vi "Subvi MultiMode Image.vi"(2 "ImageRepeatNum":u32, 3 "InFileName":string) -> (0 "ImgAbort":bool, 1 "ImgTaken":bool)   [LabVIEW 2012]
uses:
  ProSCI Global.vi
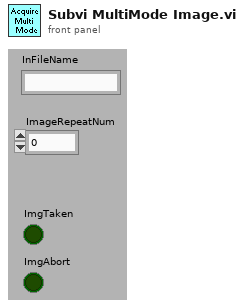
[diagram p1: front panel]
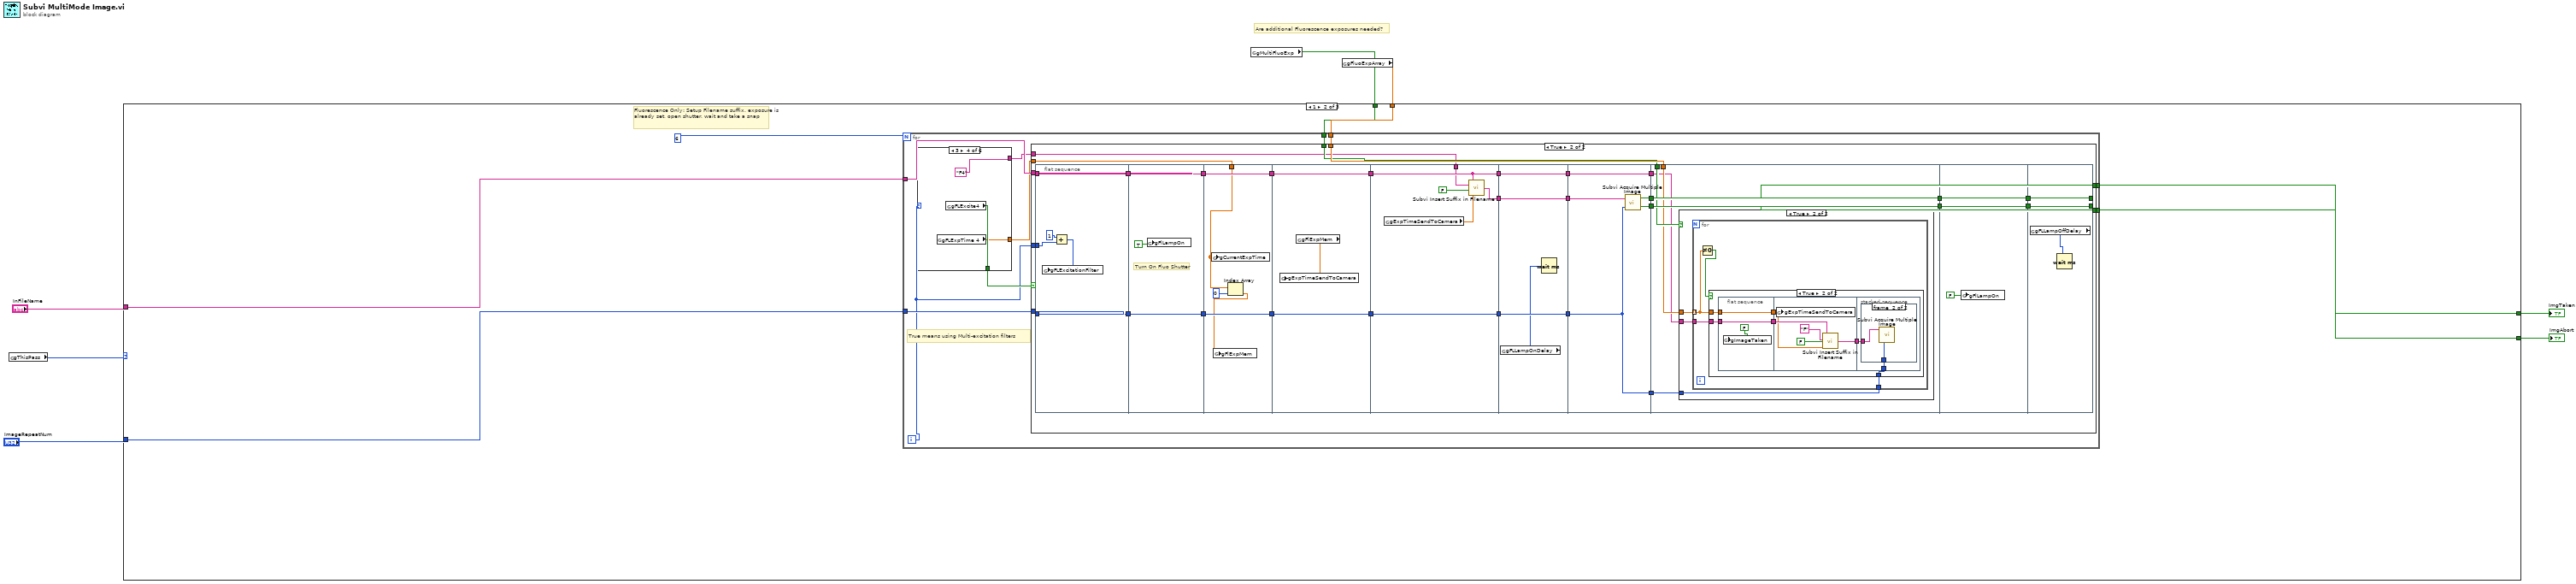
[diagram p0: block diagram]
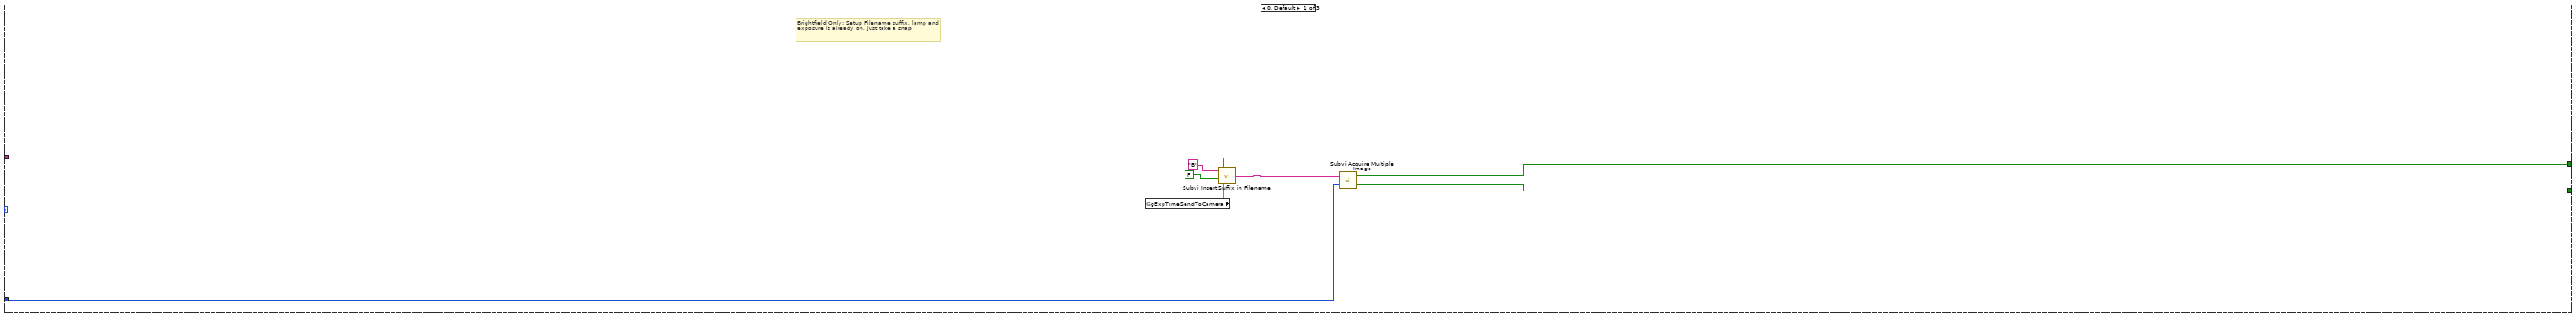
[diagram p2: hidden frame]
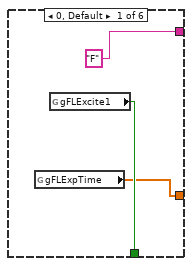
[diagram p3: hidden frame]
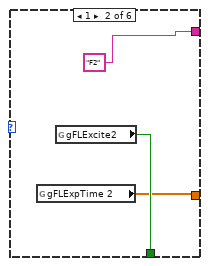
[diagram p4: hidden frame]
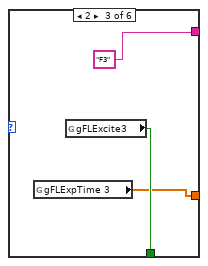
[diagram p5: hidden frame]
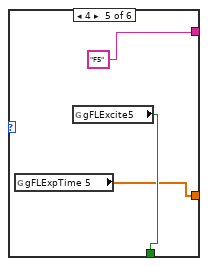
[diagram p6: hidden frame]
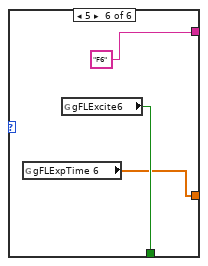
[diagram p7: hidden frame]
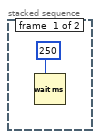
[diagram p11: hidden frame]
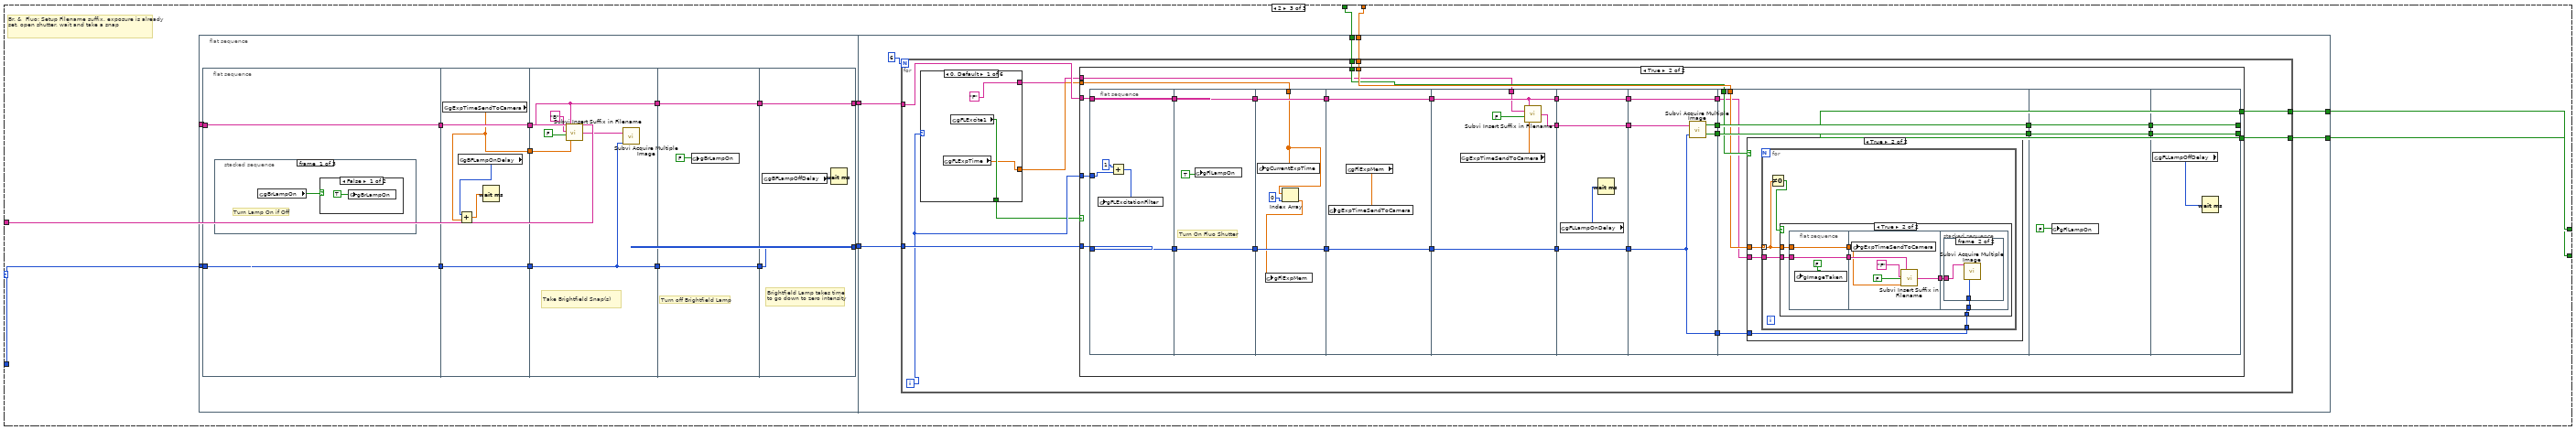
[diagram p12: hidden frame]
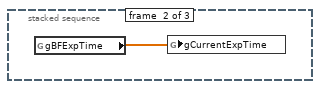
[diagram p14: hidden frame]
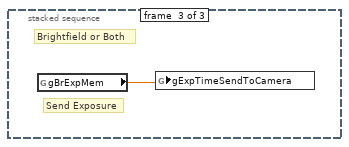
[diagram p15: hidden frame]
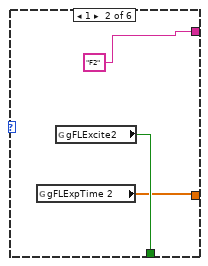
[diagram p16: hidden frame]
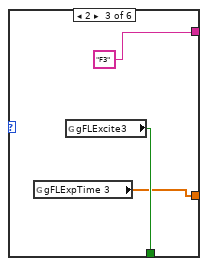
[diagram p17: hidden frame]
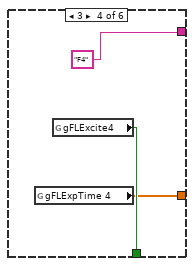
[diagram p18: hidden frame]
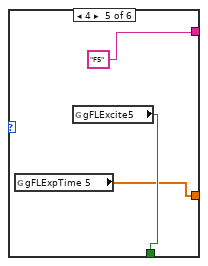
[diagram p19: hidden frame]
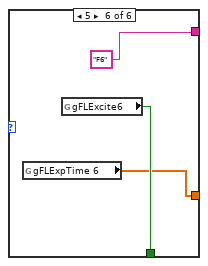
[diagram p20: hidden frame]
diagram:
  # "Are additional Fluorescence exposures needed?"
  n1 = global read "ProSCI Global.vi" "gThisPass"() -> (w3:u16)
  n2 = global read "ProSCI Global.vi" "gMultiFluoExp"() -> (w2:bool)
  n3 = global read "ProSCI Global.vi" "gFluoExpArray"() -> (w1:dbl[])
  n4 = case shown="1" w3 {
    tunnel: "InFileName" -> [w15 w18 w158]
    tunnel: "ImageRepeatNum" -> [w13 w17 w157]
    tunnel: [w12 w20 w152] -> w5
    tunnel: [w11 w19 w151] -> w4
    tunnel: w2 -> [_ w21 w156]
    tunnel: w1 -> [_ w22 w155]
    frame 0, Default {
      # "Brightfield Only: Setup Filename suffix, lamp and exposure is already on, just take a snap"
      n5 = global read "ProSCI Global.vi" "gExpTimeSendToCamera"() -> (w8:dbl)
      n6 = call "Subvi Insert Suffix in Filename.vi"("Exposure"=w8, "OnlyROI"=FALSE, "Suffix"="B" ("string"), "InFileName"=w15) -> ("OutFileName"=w14:string)
      n7 = call "Subvi Acquire Multiple Image.vi"("ImageRepeatNum"=w13, "InFileName"=w14) -> ("ImgAbort"=w11:bool, "ImgTaken"=w12:bool)
    }
    frame 1 {
      # "Fluorescence Only: Setup Filename suffix, exposure is already set, open shutter, wait and take a snap"
      n8 = for {
        N: 6 -> [_]
        tunnel: w17 -> [w31]
        tunnel: w18 -> [w30]
        tunnel: w22 -> [w29]
        tunnel: w21 -> [w28]
        tunnel: [w27] -> w20
        tunnel: [w26] -> w19
        i -> [w25]
        # "True means using Multi-excitation filters"
        n9 = case shown="3" w25 {
          tunnel: [w35 w38 w41 w44 w47 w50] -> w32
          tunnel: ["F" ("string") "F2" ("string") "F3" ("string") "F4" ("string") "F5" ("string") "F6" ("string")] -> w24
          tunnel: [w33 w36 w39 w42 w45 w48] -> w23
          frame 0, Default {
            n10 = global read "ProSCI Global.vi" "gFLExpTime"() -> (w33:dbl[])
            n11 = global read "ProSCI Global.vi" "gFLExcite1"() -> (w35:bool)
          }
          frame 1 {
            n12 = global read "ProSCI Global.vi" "gFLExpTime 2"() -> (w36:dbl[])
            n13 = global read "ProSCI Global.vi" "gFLExcite2"() -> (w38:bool)
          }
          frame 2 {
            n14 = global read "ProSCI Global.vi" "gFLExpTime 3"() -> (w39:dbl[])
            n15 = global read "ProSCI Global.vi" "gFLExcite3"() -> (w41:bool)
          }
          frame 3 {
            n16 = global read "ProSCI Global.vi" "gFLExpTime 4"() -> (w42:dbl[])
            n17 = global read "ProSCI Global.vi" "gFLExcite4"() -> (w44:bool)
          }
          frame 4 {
            n18 = global read "ProSCI Global.vi" "gFLExpTime 5"() -> (w45:dbl[])
            n19 = global read "ProSCI Global.vi" "gFLExcite5"() -> (w47:bool)
          }
          frame 5 {
            n20 = global read "ProSCI Global.vi" "gFLExpTime 6"() -> (w48:dbl[])
            n21 = global read "ProSCI Global.vi" "gFLExcite6"() -> (w50:bool)
          }
        }
        n22 = case shown="True" w32 {
          tunnel: w31 -> [_ w71]
          tunnel: w30 -> [_ w70]
          tunnel: w29 -> [_ w69]
          tunnel: w28 -> [_ w68]
          tunnel: [_ w66] -> w27
          tunnel: [_ w67] -> w26
          tunnel: w25 -> [_ w61]
          tunnel: w24 -> [_ w60]
          tunnel: w23 -> [_ w51]
          frame False {
          }
          frame True {
            n23 = flat-sequence {
              tunnel: w71 -> [w85]
              tunnel: w70 -> [w86]
              tunnel: [w86] -> w63
              tunnel: [w85] -> w62
              tunnel: w61 -> [w83]
              tunnel: [w89] -> w55
              tunnel: [w88] -> w53
              tunnel: w63 -> [w89]
              tunnel: w62 -> [w88]
              tunnel: w55 -> [w94]
              tunnel: [w94] -> w54
              tunnel: w53 -> [w93]
              tunnel: [w93] -> w52
              tunnel: w51 -> [w92]
              tunnel: [w97] -> w65
              tunnel: [w96] -> w64
              tunnel: w54 -> [w97]
              tunnel: w52 -> [w96]
              tunnel: [w103] -> w81
              tunnel: [w102] -> w80
              tunnel: [w100] -> w79
              tunnel: w65 -> [w100]
              tunnel: w64 -> [w102]
              tunnel: w60 -> [w99]
              tunnel: w81 -> [w107]
              tunnel: [w107] -> w78
              tunnel: [w106] -> w77
              tunnel: w80 -> [w106]
              tunnel: [w105] -> w76
              tunnel: w79 -> [w105]
              tunnel: w78 -> [w112]
              tunnel: w77 -> [w108]
              tunnel: [w111] -> w75
              tunnel: [w110] -> w74
              tunnel: [w109] -> w73
              tunnel: w76 -> [w109]
              tunnel: [w108] -> w72
              tunnel: w75 -> [w118]
              tunnel: [w118] -> w57
              tunnel: w74 -> [w117]
              tunnel: [w117] -> w56
              tunnel: w68 -> [w116]
              tunnel: w69 -> [w115]
              tunnel: w73 -> [w114]
              tunnel: w72 -> [w113]
              tunnel: w57 -> [w147]
              tunnel: w56 -> [w146]
              tunnel: [w147] -> w59
              tunnel: [w146] -> w58
              tunnel: [w149] -> w67
              tunnel: [w150] -> w66
              tunnel: w59 -> [w150]
              tunnel: w58 -> [w149]
              frame #0 {
                n24 = Add(x=1, y=w83) -> (x+y=w82:i32)
                n25 = global write "ProSCI Global.vi" "gFLExcitationFilter"(w82) -> ()
              }
              frame #1 {
                # "Turn On Fluo Shutter"
                n26 = global write "ProSCI Global.vi" "gFlLampOn"(TRUE ("gBrLampOn")) -> ()
              }
              frame #2 {
                n27 = global write "ProSCI Global.vi" "gCurrentExpTime"(w92) -> ()
                n28 = Index Array(array=w92, index=0) -> (element=w91:dbl)
                n29 = global write "ProSCI Global.vi" "gFlExpMem"(w91) -> ()
              }
              frame #3 {
                n30 = global read "ProSCI Global.vi" "gFlExpMem"() -> (w95:dbl)
                n31 = global write "ProSCI Global.vi" "gExpTimeSendToCamera"(w95) -> ()
              }
              frame #4 {
                n32 = global read "ProSCI Global.vi" "gExpTimeSendToCamera"() -> (w98:dbl)
                n33 = call "Subvi Insert Suffix in Filename.vi"("Exposure"=w98, "OnlyROI"=FALSE, "Suffix"=w99, "InFileName"=w100) -> ("OutFileName"=w103:string)
              }
              frame #5 {
                n34 = global read "ProSCI Global.vi" "gFLLampOnDelay"() -> (w104:i32)
                n35 = Wait (ms)(milliseconds to wait=w104) -> ()  [unwired: 1 out]
              }
              frame #6 {
                n36 = call "Subvi Acquire Multiple Image.vi"("ImageRepeatNum"=w108, "InFileName"=w112) -> ("ImgAbort"=w110:bool, "ImgTaken"=w111:bool)
              }
              frame #7 {
                n37 = case shown="True" w116 {
                  tunnel: w115 -> [_ w121]
                  tunnel: w114 -> [_ w120]
                  tunnel: w113 -> [_ w119]
                  frame False {
                  }
                  frame True {
                    n38 = for {
                      tunnel: w121 -> [w123] mode=indexing
                      tunnel: w120 -> [w125]
                      tunnel: w119 -> [w124]
                      n39 = Not Equal To 0?(x=w123) -> (x != 0?=w122:bool)
                      n40 = case shown="True" w122 {
                        tunnel: w123 -> [_ w128]
                        tunnel: w125 -> [_ w127]
                        tunnel: w124 -> [_ w126]
                        frame False {
                        }
                        frame True {
                          n41 = flat-sequence {
                            tunnel: [w133] -> w131
                            tunnel: w128 -> [w133]
                            tunnel: [w132] -> w130
                            tunnel: w127 -> [w132]
                            tunnel: w131 -> [w136]
                            tunnel: w130 -> [w137]
                            tunnel: [w135] -> w129
                            tunnel: w129 -> [w141]
                            tunnel: w126 -> [w140]
                            frame #0 {
                              n42 = global write "ProSCI Global.vi" "gImageTaken"(FALSE ("gBrLampOn")) -> ()
                            }
                            frame #1 {
                              n43 = global write "ProSCI Global.vi" "gExpTimeSendToCamera"(w136) -> ()
                              n44 = call "Subvi Insert Suffix in Filename.vi"("Exposure"=w136, "OnlyROI"=FALSE, "Suffix"="F" ("string"), "InFileName"=w137) -> ("OutFileName"=w135:string)
                            }
                            frame #2 {
                              n45 = stacked-sequence {
                                tunnel: w141 -> [_ w144]
                                tunnel: w140 -> [_ w143]
                                frame #0 {
                                n46 = Wait (ms)(milliseconds to wait=u32 250) -> ()  [unwired: 1 out]
                                }
                                frame #1 {
                                n47 = call "Subvi Acquire Multiple Image.vi"("ImageRepeatNum"=w143, "InFileName"=w144) -> ()  [unwired: 2 out]
                                }
                              }
                            }
                          }
                        }
                      }
                    }
                  }
                }
              }
              frame #8 {
                n48 = global write "ProSCI Global.vi" "gFlLampOn"(FALSE ("gBrLampOn")) -> ()
              }
              frame #9 {
                n49 = global read "ProSCI Global.vi" "gFLLampOffDelay"() -> (w148:i32)
                n50 = Wait (ms)(milliseconds to wait=w148) -> ()  [unwired: 1 out]
              }
            }
          }
        }
      }
    }
    frame 2 {
      # "Br. &  Fluo: Setup Filename suffix, exposure is already set, open shutter, wait and take a snap"
      n51 = flat-sequence {
        tunnel: w158 -> [w169]
        tunnel: w157 -> [w168]
        tunnel: [w167] -> w154
        tunnel: [w166] -> w153
        tunnel: w156 -> [w200]
        tunnel: w155 -> [w199]
        tunnel: w154 -> [w198]
        tunnel: w153 -> [w197]
        tunnel: [w196] -> w152
        tunnel: [w195] -> w151
        frame #0 {
          n52 = flat-sequence {
            tunnel: w168 -> [w172]
            tunnel: w169 -> [w173]
            tunnel: [w173] -> w163
            tunnel: [w172] -> w161
            tunnel: w163 -> [w182]
            tunnel: [w182] -> w162
            tunnel: w161 -> [w181]
            tunnel: [w181] -> w160
            tunnel: [w178] -> w159
            tunnel: [w186] -> w165
            tunnel: [w185] -> w164
            tunnel: w162 -> [w185]
            tunnel: w160 -> [w186]
            tunnel: w159 -> [w183]
            tunnel: w165 -> [w191]
            tunnel: [w191] -> w171
            tunnel: w164 -> [w190]
            tunnel: [w190] -> w170
            tunnel: w171 -> [w192]
            tunnel: w170 -> [w193]
            tunnel: [w193] -> w167
            tunnel: [w192] -> w166
            frame #0 {
              n53 = stacked-sequence {
                frame #0 {
                  # "Turn Lamp On if Off"
                  n54 = global read "ProSCI Global.vi" "gBrLampOn"() -> (w174:bool)
                  n55 = case shown="False" w174 {
                    frame False {
                      n56 = global write "ProSCI Global.vi" "gBrLampOn"(TRUE ("gBrLampOn")) -> ()
                    }
                    frame True {
                    }
                  }
                }
                frame #1 {
                  n57 = global read "ProSCI Global.vi" "gBFExpTime"() -> (w176:dbl[])
                  n58 = global write "ProSCI Global.vi" "gCurrentExpTime"(w176) -> ()
                }
                frame #2 {
                  # "Send Exposure"
                  # "Brightfield or Both"
                  n59 = global read "ProSCI Global.vi" "gBrExpMem"() -> (w177:dbl)
                  n60 = global write "ProSCI Global.vi" "gExpTimeSendToCamera"(w177) -> ()
                }
              }
            }
            frame #1 {
              n61 = global read "ProSCI Global.vi" "gExpTimeSendToCamera"() -> (w178:dbl)
              n62 = global read "ProSCI Global.vi" "gBFLampOnDelay"() -> (w180:i32)
              n63 = Add(x=w180, y=w178) -> (x+y=w179:dbl)
              n64 = Wait (ms)(milliseconds to wait=w179) -> ()  [unwired: 1 out]
            }
            frame #2 {
              # "Take Brightfield Snap(s)"
              n65 = call "Subvi Insert Suffix in Filename.vi"("Exposure"=w183, "OnlyROI"=FALSE, "Suffix"="B" ("string"), "InFileName"=w185) -> ("OutFileName"=w187:string)
              n66 = call "Subvi Acquire Multiple Image.vi"("ImageRepeatNum"=w186, "InFileName"=w187) -> ()  [unwired: 2 out]
            }
            frame #3 {
              # "Turn off Brightfield Lamp"
              n67 = global write "ProSCI Global.vi" "gBrLampOn"(FALSE ("gBrLampOn")) -> ()
            }
            frame #4 {
              # "Brightfield Lamp takes time to go down to zero intensity"
              n68 = global read "ProSCI Global.vi" "gBFLampOffDelay"() -> (w194:i32)
              n69 = Wait (ms)(milliseconds to wait=w194) -> ()  [unwired: 1 out]
            }
          }
        }
        frame #1 {
          n70 = for {
            N: 6 -> [_]
            tunnel: w197 -> [w211]
            tunnel: w198 -> [w210]
            tunnel: w199 -> [w209]
            tunnel: w200 -> [w208]
            tunnel: [w207] -> w196
            tunnel: [w206] -> w195
            i -> [w204]
            n71 = case shown="0, Default" w204 {
              tunnel: [w214 w217 w220 w223 w226 w229] -> w203
              tunnel: ["F" ("string") "F2" ("string") "F3" ("string") "F4" ("string") "F5" ("string") "F6" ("string")] -> w202
              tunnel: [w212 w215 w218 w221 w224 w227] -> w205
              frame 0, Default {
                n72 = global read "ProSCI Global.vi" "gFLExpTime"() -> (w212:dbl[])
                n73 = global read "ProSCI Global.vi" "gFLExcite1"() -> (w214:bool)
              }
              frame 1 {
                n74 = global read "ProSCI Global.vi" "gFLExpTime 2"() -> (w215:dbl[])
                n75 = global read "ProSCI Global.vi" "gFLExcite2"() -> (w217:bool)
              }
              frame 2 {
                n76 = global read "ProSCI Global.vi" "gFLExpTime 3"() -> (w218:dbl[])
                n77 = global read "ProSCI Global.vi" "gFLExcite3"() -> (w220:bool)
              }
              frame 3 {
                n78 = global read "ProSCI Global.vi" "gFLExpTime 4"() -> (w221:dbl[])
                n79 = global read "ProSCI Global.vi" "gFLExcite4"() -> (w223:bool)
              }
              frame 4 {
                n80 = global read "ProSCI Global.vi" "gFLExpTime 5"() -> (w224:dbl[])
                n81 = global read "ProSCI Global.vi" "gFLExcite5"() -> (w226:bool)
              }
              frame 5 {
                n82 = global read "ProSCI Global.vi" "gFLExpTime 6"() -> (w227:dbl[])
                n83 = global read "ProSCI Global.vi" "gFLExcite6"() -> (w229:bool)
              }
            }
            n84 = case shown="True" w203 {
              tunnel: w211 -> [_ w250]
              tunnel: w210 -> [_ w249]
              tunnel: w209 -> [_ w248]
              tunnel: w208 -> [_ w247]
              tunnel: [_ w245] -> w207
              tunnel: [_ w246] -> w206
              tunnel: w204 -> [_ w240]
              tunnel: w202 -> [_ w239]
              tunnel: w205 -> [_ w230]
              frame False {
              }
              frame True {
                n85 = flat-sequence {
                  tunnel: w250 -> [w264]
                  tunnel: w249 -> [w265]
                  tunnel: [w265] -> w242
                  tunnel: [w264] -> w241
                  tunnel: w240 -> [w262]
                  tunnel: [w268] -> w234
                  tunnel: [w267] -> w232
                  tunnel: w242 -> [w268]
                  tunnel: w241 -> [w267]
                  tunnel: w234 -> [w273]
                  tunnel: [w273] -> w233
                  tunnel: w232 -> [w272]
                  tunnel: [w272] -> w231
                  tunnel: w230 -> [w271]
                  tunnel: [w276] -> w244
                  tunnel: [w275] -> w243
                  tunnel: w233 -> [w276]
                  tunnel: w231 -> [w275]
                  tunnel: [w282] -> w260
                  tunnel: [w281] -> w259
                  tunnel: [w279] -> w258
                  tunnel: w244 -> [w279]
                  tunnel: w243 -> [w281]
                  tunnel: w239 -> [w278]
                  tunnel: w260 -> [w286]
                  tunnel: [w286] -> w257
                  tunnel: [w285] -> w256
                  tunnel: w259 -> [w285]
                  tunnel: [w284] -> w255
                  tunnel: w258 -> [w284]
                  tunnel: w257 -> [w291]
                  tunnel: w256 -> [w287]
                  tunnel: [w290] -> w254
                  tunnel: [w289] -> w253
                  tunnel: [w288] -> w252
                  tunnel: w255 -> [w288]
                  tunnel: [w287] -> w251
                  tunnel: w254 -> [w297]
                  tunnel: [w297] -> w236
                  tunnel: w253 -> [w296]
                  tunnel: [w296] -> w235
                  tunnel: w247 -> [w295]
                  tunnel: w248 -> [w294]
                  tunnel: w252 -> [w293]
                  tunnel: w251 -> [w292]
                  tunnel: w236 -> [w326]
                  tunnel: w235 -> [w325]
                  tunnel: [w326] -> w238
                  tunnel: [w325] -> w237
                  tunnel: [w328] -> w246
                  tunnel: [w329] -> w245
                  tunnel: w238 -> [w329]
                  tunnel: w237 -> [w328]
                  frame #0 {
                    n86 = Add(x=1, y=w262) -> (x+y=w261:i32)
                    n87 = global write "ProSCI Global.vi" "gFLExcitationFilter"(w261) -> ()
                  }
                  frame #1 {
                    # "Turn On Fluo Shutter"
                    n88 = global write "ProSCI Global.vi" "gFlLampOn"(TRUE ("gBrLampOn")) -> ()
                  }
                  frame #2 {
                    n89 = global write "ProSCI Global.vi" "gCurrentExpTime"(w271) -> ()
                    n90 = Index Array(array=w271, index=0) -> (element=w270:dbl)
                    n91 = global write "ProSCI Global.vi" "gFlExpMem"(w270) -> ()
                  }
                  frame #3 {
                    n92 = global read "ProSCI Global.vi" "gFlExpMem"() -> (w274:dbl)
                    n93 = global write "ProSCI Global.vi" "gExpTimeSendToCamera"(w274) -> ()
                  }
                  frame #4 {
                    n94 = global read "ProSCI Global.vi" "gExpTimeSendToCamera"() -> (w277:dbl)
                    n95 = call "Subvi Insert Suffix in Filename.vi"("Exposure"=w277, "OnlyROI"=FALSE, "Suffix"=w278, "InFileName"=w279) -> ("OutFileName"=w282:string)
                  }
                  frame #5 {
                    n96 = global read "ProSCI Global.vi" "gFLLampOnDelay"() -> (w283:i32)
                    n97 = Wait (ms)(milliseconds to wait=w283) -> ()  [unwired: 1 out]
                  }
                  frame #6 {
                    n98 = call "Subvi Acquire Multiple Image.vi"("ImageRepeatNum"=w287, "InFileName"=w291) -> ("ImgAbort"=w289:bool, "ImgTaken"=w290:bool)
                  }
                  frame #7 {
                    n99 = case shown="True" w295 {
                      tunnel: w294 -> [_ w300]
                      tunnel: w293 -> [_ w299]
                      tunnel: w292 -> [_ w298]
                      frame False {
                      }
                      frame True {
                        n100 = for {
                          tunnel: w300 -> [w302] mode=indexing
                          tunnel: w299 -> [w304]
                          tunnel: w298 -> [w303]
                          n101 = Not Equal To 0?(x=w302) -> (x != 0?=w301:bool)
                          n102 = case shown="True" w301 {
                            tunnel: w302 -> [_ w307]
                            tunnel: w304 -> [_ w306]
                            tunnel: w303 -> [_ w305]
                            frame False {
                            }
                            frame True {
                              n103 = flat-sequence {
                                tunnel: [w312] -> w310
                                tunnel: w307 -> [w312]
                                tunnel: [w311] -> w309
                                tunnel: w306 -> [w311]
                                tunnel: w310 -> [w315]
                                tunnel: w309 -> [w316]
                                tunnel: [w314] -> w308
                                tunnel: w308 -> [w320]
                                tunnel: w305 -> [w319]
                                frame #0 {
                                n104 = global write "ProSCI Global.vi" "gImageTaken"(FALSE ("gBrLampOn")) -> ()
                                }
                                frame #1 {
                                n105 = global write "ProSCI Global.vi" "gExpTimeSendToCamera"(w315) -> ()
                                n106 = call "Subvi Insert Suffix in Filename.vi"("Exposure"=w315, "OnlyROI"=FALSE, "Suffix"="F" ("string"), "InFileName"=w316) -> ("OutFileName"=w314:string)
                                }
                                frame #2 {
                                n107 = stacked-sequence {
                                tunnel: w320 -> [_ w323]
                                tunnel: w319 -> [_ w322]
                                frame #0 {
                                n108 = Wait (ms)(milliseconds to wait=u32 250) -> ()  [unwired: 1 out]
                                }
                                frame #1 {
                                n109 = call "Subvi Acquire Multiple Image.vi"("ImageRepeatNum"=w322, "InFileName"=w323) -> ()  [unwired: 2 out]
                                }
                                }
                                }
                              }
                            }
                          }
                        }
                      }
                    }
                  }
                  frame #8 {
                    n110 = global write "ProSCI Global.vi" "gFlLampOn"(FALSE ("gBrLampOn")) -> ()
                  }
                  frame #9 {
                    n111 = global read "ProSCI Global.vi" "gFLLampOffDelay"() -> (w327:i32)
                    n112 = Wait (ms)(milliseconds to wait=w327) -> ()  [unwired: 1 out]
                  }
                }
              }
            }
          }
        }
      }
    }
  }
  "ImgTaken" <- w5
  "ImgAbort" <- w4
